vi "pmtMean.vi"(1 "pmt counts":u32, 2 "input queue":refnum<queue>) -> (0 "mean":dbl format="%0.2f")   [LabVIEW 2012]
uses:
  My Documents/VIs/Control 1.ctl
  <vilib>/Analysis/baseanly.llb/Mean (DBL).vi
  <vilib>/Analysis/NI_AALBase.lvlib
panel:
  out "Mean":T1=45.0 format="%0.2d"
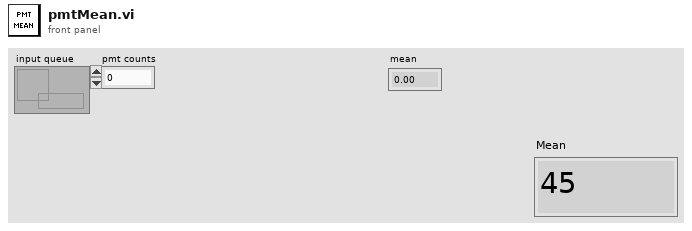
[diagram p1: front panel]
types:
  T1 = typedef "Control 1.ctl" = dbl
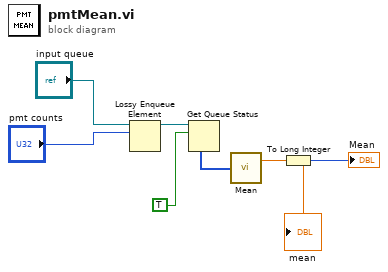
[diagram p0: block diagram]
diagram:
  n1 = Lossy Enqueue Element(queue="input queue", element="pmt counts") -> (queue out=w7:refnum<queue>)  [unwired: 1 in, 3 out]
  n2 = Get Queue Status(queue=w7, return elements? (F)=TRUE) -> (elements=w5:u32[])  [unwired: 1 in, 7 out]
  n3 = call-poly <vilib>:"Mean.vi"("X"=w5) -> ("mean"=w3:dbl)  [unwired: 1 out]
  "mean" <- w3
  n4 = To Long Integer(number=w3) -> (32bit integer=→"Mean":i32)
